vi "LC_Control.vi"() -> ()   [LabVIEW 2016]
panel:
  out "RealPowerPriority_cg 2":bool
  out "online_pb":bool
  out "enabled_pb":bool
  out "connectedtogrid_cg":bool
  out "alarmestop_cg":bool
  out "ackalarms_cg 2":bool
  out "zonesonline_cg":dbl
  out "totalrealpower_mr":dbl
  out "totalreactivepower_mr":dbl
  out "realpoweroutput_cg":dbl
  out "realpowercapacity_cg":dbl
  out "reactivepoweroutput_cg":dbl
  out "reactivepowercapacity_cg":dbl
  out "qdischargelimit_cg":dbl
  out "qchargelimit_cg":dbl
  out "powerfactor_mr":dbl
  out "pdischargelimit_cg":dbl
  out "pchargelimit_cg":dbl
  out "mintemp_bz":dbl
  out "minsoc_bz":dbl
  out "maxtemp_bz":dbl
  out "maxsoc_bz":dbl
  out "groupmode_cg":dbl
  out "frequency_mr":dbl
  out "dischargecapacity_cg":dbl
  out "commandin_rtp":dbl
  out "chargecapacity_cg":dbl
  out "avgtemp_bz":dbl
  out "averagesoc_cg":dbl
  out "averagelinevoltage_mr":dbl
  out "averagelinecurrent_mr":dbl
  out "availableenergy_cg":dbl
  in  "referenceInput_rtp":bool
  in  "referenceInput_rp":bool
  in  "modecontrol_cg":bool
  in  "ackalarms_cg":dbl
  in  "RealPowerPriority_cg":dbl
  out "LC_Error_Clear":bool
  out "LC_Vol_Ref":dbl
  out "LC_Sync_Mag_Diff":dbl
  out "LC_Sync_Freq_Diff":dbl
  out "LC_Sync_Ang_Diff":dbl
  out "LC_Status_Cmd":dbl
  out "LC_Re_Pwr_Ref":dbl
  out "LC_Pwr_Ref":dbl
  out "LC_Freq_Ref":dbl
  in  "LC_Vol":dbl
  in  "LC_Status":dbl
  in  "LC_Re_Pwr":dbl
  in  "LC_Pwr":dbl
  in  "LC_Freq":dbl
  in  "LC_Error":dbl
  in  "LC_BESS_SOC":dbl
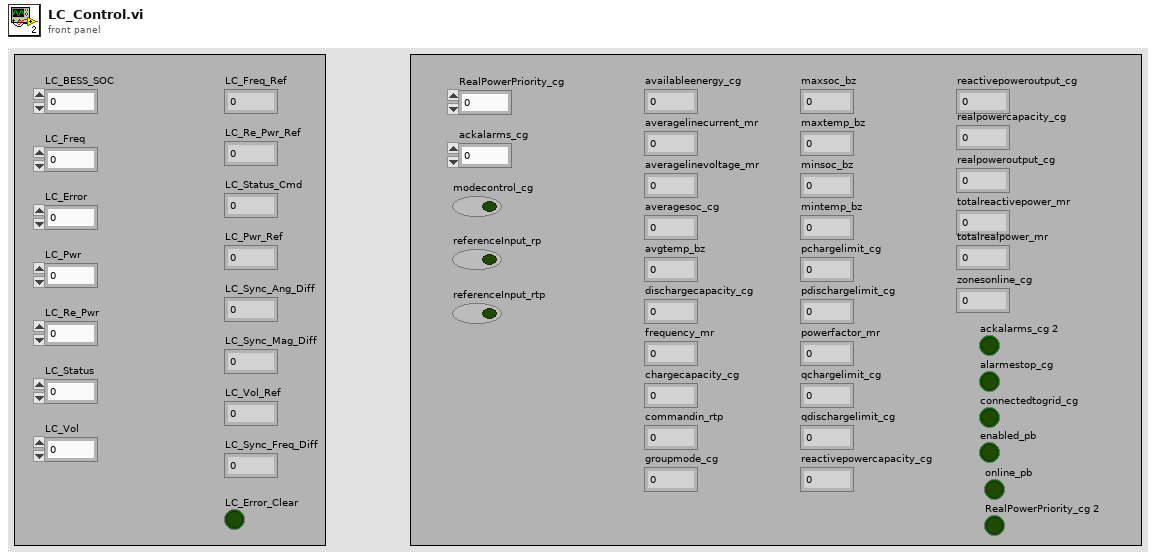
[diagram p1: front panel]
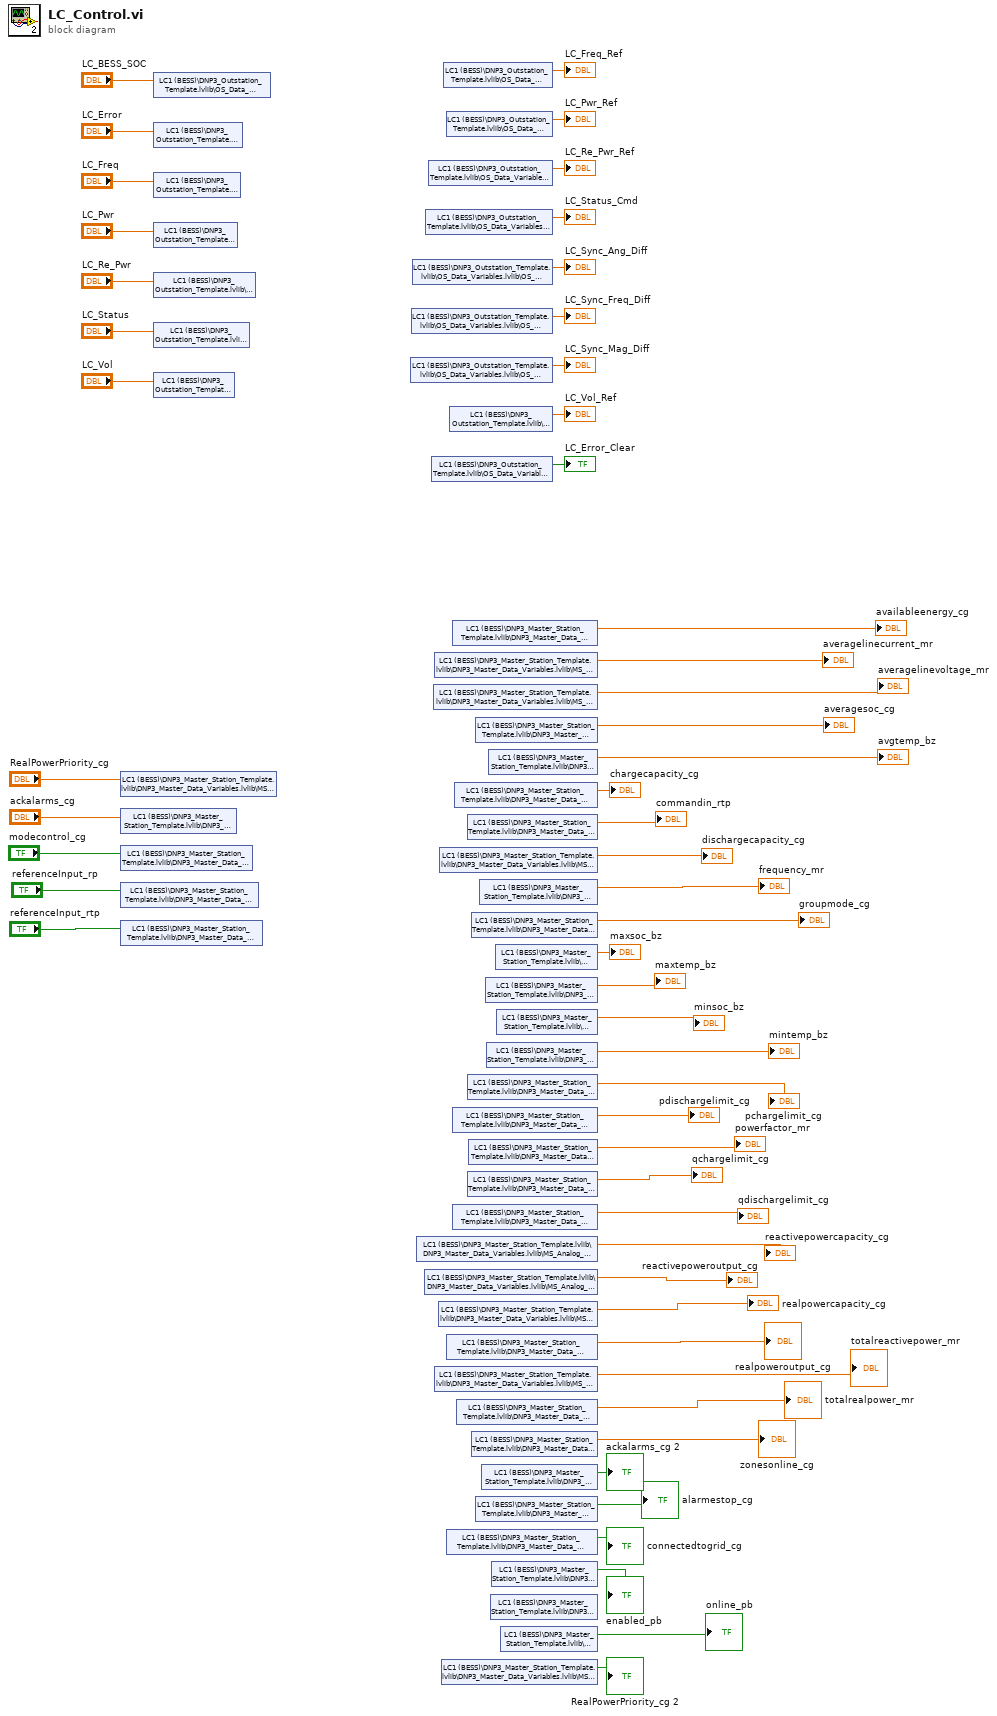
[diagram p0: block diagram]
diagram:
  n1 = shared-variable "LC1 (BESS)\\DNP3_Master_Station_Template.lvlib\\DNP3_Master_Data_Variables.lvlib\\MS_Analog_Control.lvlib\\RealPowerPriority_cg"("RealPowerPriority_cg") -> ()  [unwired: 1 in, 1 out]
  n2 = shared-variable "LC1 (BESS)\\DNP3_Master_Station_Template.lvlib\\DNP3_Master_Data_Variables.lvlib\\MS_Analog_Control.lvlib\\ackalarms_cg"("ackalarms_cg") -> ()  [unwired: 1 in, 1 out]
  n3 = shared-variable "LC1 (BESS)\\DNP3_Master_Station_Template.lvlib\\DNP3_Master_Data_Variables.lvlib\\MS_Binary_Control.lvlib\\modecontrol_cg"("modecontrol_cg") -> ()  [unwired: 1 in, 1 out]
  n4 = shared-variable "LC1 (BESS)\\DNP3_Master_Station_Template.lvlib\\DNP3_Master_Data_Variables.lvlib\\MS_Binary_Control.lvlib\\referenceInput_rp"("referenceInput_rp") -> ()  [unwired: 1 in, 1 out]
  n5 = shared-variable "LC1 (BESS)\\DNP3_Master_Station_Template.lvlib\\DNP3_Master_Data_Variables.lvlib\\MS_Binary_Control.lvlib\\referenceInput_rtp"("referenceInput_rtp") -> ()  [unwired: 1 in, 1 out]
  n6 = shared-variable "LC1 (BESS)\\DNP3_Outstation_Template.lvlib\\OS_Data_Variables.lvlib\\OS_Analog_Status.lvlib\\LC_BESS_SOC"("LC_BESS_SOC") -> ()  [unwired: 1 in, 1 out]
  n7 = shared-variable "LC1 (BESS)\\DNP3_Outstation_Template.lvlib\\OS_Data_Variables.lvlib\\OS_Analog_Status.lvlib\\LC_Error"("LC_Error") -> ()  [unwired: 1 in, 1 out]
  n8 = shared-variable "LC1 (BESS)\\DNP3_Outstation_Template.lvlib\\OS_Data_Variables.lvlib\\OS_Analog_Status.lvlib\\LC_Freq"("LC_Freq") -> ()  [unwired: 1 in, 1 out]
  n9 = shared-variable "LC1 (BESS)\\DNP3_Outstation_Template.lvlib\\OS_Data_Variables.lvlib\\OS_Analog_Status.lvlib\\LC_Pwr"("LC_Pwr") -> ()  [unwired: 1 in, 1 out]
  n10 = shared-variable "LC1 (BESS)\\DNP3_Outstation_Template.lvlib\\OS_Data_Variables.lvlib\\OS_Analog_Status.lvlib\\LC_Re_Pwr"("LC_Re_Pwr") -> ()  [unwired: 1 in, 1 out]
  n11 = shared-variable "LC1 (BESS)\\DNP3_Outstation_Template.lvlib\\OS_Data_Variables.lvlib\\OS_Analog_Status.lvlib\\LC_Status"("LC_Status") -> ()  [unwired: 1 in, 1 out]
  n12 = shared-variable "LC1 (BESS)\\DNP3_Outstation_Template.lvlib\\OS_Data_Variables.lvlib\\OS_Analog_Status.lvlib\\LC_Vol"("LC_Vol") -> ()  [unwired: 1 in, 1 out]
  n13 = shared-variable "LC1 (BESS)\\DNP3_Outstation_Template.lvlib\\OS_Data_Variables.lvlib\\OS_Analog_Control.lvlib\\LC_Sync_Mag_Diff"() -> (→"LC_Sync_Mag_Diff":dbl)  [unwired: 1 in, 1 out]
  n14 = shared-variable "LC1 (BESS)\\DNP3_Outstation_Template.lvlib\\OS_Data_Variables.lvlib\\OS_Analog_Control.lvlib\\LC_Sync_Freq_Diff"() -> (→"LC_Sync_Freq_Diff":dbl)  [unwired: 1 in, 1 out]
  n15 = shared-variable "LC1 (BESS)\\DNP3_Outstation_Template.lvlib\\OS_Data_Variables.lvlib\\OS_Analog_Control.lvlib\\LC_Sync_Ang_Diff"() -> (→"LC_Sync_Ang_Diff":dbl)  [unwired: 1 in, 1 out]
  n16 = shared-variable "LC1 (BESS)\\DNP3_Master_Station_Template.lvlib\\DNP3_Master_Data_Variables.lvlib\\MS_Analog_Status.lvlib\\reactivepowercapacity_cg"() -> (→"reactivepowercapacity_cg":dbl)  [unwired: 1 in, 1 out]
  n17 = shared-variable "LC1 (BESS)\\DNP3_Master_Station_Template.lvlib\\DNP3_Master_Data_Variables.lvlib\\MS_Analog_Status.lvlib\\reactivepoweroutput_cg"() -> (→"reactivepoweroutput_cg":dbl)  [unwired: 1 in, 1 out]
  n18 = shared-variable "LC1 (BESS)\\DNP3_Outstation_Template.lvlib\\OS_Data_Variables.lvlib\\OS_Analog_Control.lvlib\\LC_Status_Cmd"() -> (→"LC_Status_Cmd":dbl)  [unwired: 1 in, 1 out]
  n19 = shared-variable "LC1 (BESS)\\DNP3_Outstation_Template.lvlib\\OS_Data_Variables.lvlib\\OS_Analog_Control.lvlib\\LC_Re_Pwr_Ref"() -> (→"LC_Re_Pwr_Ref":dbl)  [unwired: 1 in, 1 out]
  n20 = shared-variable "LC1 (BESS)\\DNP3_Outstation_Template.lvlib\\OS_Data_Variables.lvlib\\OS_Binary_Control.lvlib\\LC_Error_Clear"() -> (→"LC_Error_Clear":bool)  [unwired: 1 in, 1 out]
  n21 = shared-variable "LC1 (BESS)\\DNP3_Master_Station_Template.lvlib\\DNP3_Master_Data_Variables.lvlib\\MS_Analog_Status.lvlib\\averagelinevoltage_mr"() -> (→"averagelinevoltage_mr":dbl)  [unwired: 1 in, 1 out]
  n22 = shared-variable "LC1 (BESS)\\DNP3_Master_Station_Template.lvlib\\DNP3_Master_Data_Variables.lvlib\\MS_Analog_Status.lvlib\\averagelinecurrent_mr"() -> (→"averagelinecurrent_mr":dbl)  [unwired: 1 in, 1 out]
  n23 = shared-variable "LC1 (BESS)\\DNP3_Master_Station_Template.lvlib\\DNP3_Master_Data_Variables.lvlib\\MS_Analog_Status.lvlib\\totalreactivepower_mr"() -> (→"totalreactivepower_mr":dbl)  [unwired: 1 in, 1 out]
  n24 = shared-variable "LC1 (BESS)\\DNP3_Master_Station_Template.lvlib\\DNP3_Master_Data_Variables.lvlib\\MS_Analog_Status.lvlib\\realpowercapacity_cg"() -> (→"realpowercapacity_cg":dbl)  [unwired: 1 in, 1 out]
  n25 = shared-variable "LC1 (BESS)\\DNP3_Master_Station_Template.lvlib\\DNP3_Master_Data_Variables.lvlib\\MS_Analog_Status.lvlib\\dischargecapacity_cg"() -> (→"dischargecapacity_cg":dbl)  [unwired: 1 in, 1 out]
  n26 = shared-variable "LC1 (BESS)\\DNP3_Master_Station_Template.lvlib\\DNP3_Master_Data_Variables.lvlib\\MS_Binary_Status.lvlib\\RealPowerPriority_cg"() -> (→"RealPowerPriority_cg 2":bool)  [unwired: 1 in, 1 out]
  n27 = shared-variable "LC1 (BESS)\\DNP3_Outstation_Template.lvlib\\OS_Data_Variables.lvlib\\OS_Analog_Control.lvlib\\LC_Freq_Ref"() -> (→"LC_Freq_Ref":dbl)  [unwired: 1 in, 1 out]
  n28 = shared-variable "LC1 (BESS)\\DNP3_Outstation_Template.lvlib\\OS_Data_Variables.lvlib\\OS_Analog_Control.lvlib\\LC_Pwr_Ref"() -> (→"LC_Pwr_Ref":dbl)  [unwired: 1 in, 1 out]
  n29 = shared-variable "LC1 (BESS)\\DNP3_Master_Station_Template.lvlib\\DNP3_Master_Data_Variables.lvlib\\MS_Analog_Status.lvlib\\realpoweroutput_cg"() -> (→"realpoweroutput_cg":dbl)  [unwired: 1 in, 1 out]
  n30 = shared-variable "LC1 (BESS)\\DNP3_Master_Station_Template.lvlib\\DNP3_Master_Data_Variables.lvlib\\MS_Binary_Status.lvlib\\connectedtogrid_cg"() -> (→"connectedtogrid_cg":bool)  [unwired: 1 in, 1 out]
  n31 = shared-variable "LC1 (BESS)\\DNP3_Outstation_Template.lvlib\\OS_Data_Variables.lvlib\\OS_Analog_Control.lvlib\\LC_Vol_Ref"() -> (→"LC_Vol_Ref":dbl)  [unwired: 1 in, 1 out]
  n32 = shared-variable "LC1 (BESS)\\DNP3_Master_Station_Template.lvlib\\DNP3_Master_Data_Variables.lvlib\\MS_Analog_Status.lvlib\\availableenergy_cg"() -> (→"availableenergy_cg":dbl)  [unwired: 1 in, 1 out]
  n33 = shared-variable "LC1 (BESS)\\DNP3_Master_Station_Template.lvlib\\DNP3_Master_Data_Variables.lvlib\\MS_Analog_Status.lvlib\\pdischargelimit_cg"() -> (→"pdischargelimit_cg":dbl)  [unwired: 1 in, 1 out]
  n34 = shared-variable "LC1 (BESS)\\DNP3_Master_Station_Template.lvlib\\DNP3_Master_Data_Variables.lvlib\\MS_Analog_Status.lvlib\\qdischargelimit_cg"() -> (→"qdischargelimit_cg":dbl)  [unwired: 1 in, 1 out]
  n35 = shared-variable "LC1 (BESS)\\DNP3_Master_Station_Template.lvlib\\DNP3_Master_Data_Variables.lvlib\\MS_Analog_Status.lvlib\\chargecapacity_cg"() -> (→"chargecapacity_cg":dbl)  [unwired: 1 in, 1 out]
  n36 = shared-variable "LC1 (BESS)\\DNP3_Master_Station_Template.lvlib\\DNP3_Master_Data_Variables.lvlib\\MS_Analog_Status.lvlib\\totalrealpower_mr"() -> (→"totalrealpower_mr":dbl)  [unwired: 1 in, 1 out]
  n37 = shared-variable "LC1 (BESS)\\DNP3_Master_Station_Template.lvlib\\DNP3_Master_Data_Variables.lvlib\\MS_Analog_Status.lvlib\\commandin_rtp"() -> (→"commandin_rtp":dbl)  [unwired: 1 in, 1 out]
  n38 = shared-variable "LC1 (BESS)\\DNP3_Master_Station_Template.lvlib\\DNP3_Master_Data_Variables.lvlib\\MS_Analog_Status.lvlib\\pchargelimit_cg"() -> (→"pchargelimit_cg":dbl)  [unwired: 1 in, 1 out]
  n39 = shared-variable "LC1 (BESS)\\DNP3_Master_Station_Template.lvlib\\DNP3_Master_Data_Variables.lvlib\\MS_Analog_Status.lvlib\\qchargelimit_cg"() -> (→"qchargelimit_cg":dbl)  [unwired: 1 in, 1 out]
  n40 = shared-variable "LC1 (BESS)\\DNP3_Master_Station_Template.lvlib\\DNP3_Master_Data_Variables.lvlib\\MS_Analog_Status.lvlib\\powerfactor_mr"() -> (→"powerfactor_mr":dbl)  [unwired: 1 in, 1 out]
  n41 = shared-variable "LC1 (BESS)\\DNP3_Master_Station_Template.lvlib\\DNP3_Master_Data_Variables.lvlib\\MS_Analog_Status.lvlib\\groupmode_cg"() -> (→"groupmode_cg":dbl)  [unwired: 1 in, 1 out]
  n42 = shared-variable "LC1 (BESS)\\DNP3_Master_Station_Template.lvlib\\DNP3_Master_Data_Variables.lvlib\\MS_Analog_Status.lvlib\\zonesonline_cg"() -> (→"zonesonline_cg":dbl)  [unwired: 1 in, 1 out]
  n43 = shared-variable "LC1 (BESS)\\DNP3_Master_Station_Template.lvlib\\DNP3_Master_Data_Variables.lvlib\\MS_Analog_Status.lvlib\\averagesoc_cg"() -> (→"averagesoc_cg":dbl)  [unwired: 1 in, 1 out]
  n44 = shared-variable "LC1 (BESS)\\DNP3_Master_Station_Template.lvlib\\DNP3_Master_Data_Variables.lvlib\\MS_Binary_Status.lvlib\\alarmestop_cg"() -> (→"alarmestop_cg":bool)  [unwired: 1 in, 1 out]
  n45 = shared-variable "LC1 (BESS)\\DNP3_Master_Station_Template.lvlib\\DNP3_Master_Data_Variables.lvlib\\MS_Analog_Status.lvlib\\frequency_mr"() -> (→"frequency_mr":dbl)  [unwired: 1 in, 1 out]
  n46 = shared-variable "LC1 (BESS)\\DNP3_Master_Station_Template.lvlib\\DNP3_Master_Data_Variables.lvlib\\MS_Binary_Status.lvlib\\ackalarms_cg"() -> (→"ackalarms_cg 2":bool)  [unwired: 1 in, 1 out]
  n47 = shared-variable "LC1 (BESS)\\DNP3_Master_Station_Template.lvlib\\DNP3_Master_Data_Variables.lvlib\\MS_Analog_Status.lvlib\\maxtemp_bz"() -> (→"maxtemp_bz":dbl)  [unwired: 1 in, 1 out]
  n48 = shared-variable "LC1 (BESS)\\DNP3_Master_Station_Template.lvlib\\DNP3_Master_Data_Variables.lvlib\\MS_Analog_Status.lvlib\\mintemp_bz"() -> (→"mintemp_bz":dbl)  [unwired: 1 in, 1 out]
  n49 = shared-variable "LC1 (BESS)\\DNP3_Master_Station_Template.lvlib\\DNP3_Master_Data_Variables.lvlib\\MS_Analog_Status.lvlib\\avgtemp_bz"() -> (→"avgtemp_bz":dbl)  [unwired: 1 in, 1 out]
  n50 = shared-variable "LC1 (BESS)\\DNP3_Master_Station_Template.lvlib\\DNP3_Master_Data_Variables.lvlib\\MS_Binary_Status.lvlib\\enabled_rtp"() -> ()  [unwired: 1 in, 2 out]
  n51 = shared-variable "LC1 (BESS)\\DNP3_Master_Station_Template.lvlib\\DNP3_Master_Data_Variables.lvlib\\MS_Binary_Status.lvlib\\enabled_pb"() -> (→"enabled_pb":bool)  [unwired: 1 in, 1 out]
  n52 = shared-variable "LC1 (BESS)\\DNP3_Master_Station_Template.lvlib\\DNP3_Master_Data_Variables.lvlib\\MS_Analog_Status.lvlib\\maxsoc_bz"() -> (→"maxsoc_bz":dbl)  [unwired: 1 in, 1 out]
  n53 = shared-variable "LC1 (BESS)\\DNP3_Master_Station_Template.lvlib\\DNP3_Master_Data_Variables.lvlib\\MS_Analog_Status.lvlib\\minsoc_bz"() -> (→"minsoc_bz":dbl)  [unwired: 1 in, 1 out]
  n54 = shared-variable "LC1 (BESS)\\DNP3_Master_Station_Template.lvlib\\DNP3_Master_Data_Variables.lvlib\\MS_Binary_Status.lvlib\\online_pb"() -> (→"online_pb":bool)  [unwired: 1 in, 1 out]
